vi "Update time schedule.vi"   [LabVIEW 2020]
uses:
  <vilib>/Utility/miscctls.llb/LVDateTimeRec.ctl
  Global variable.vi
types:
  T1 = typedef "LVDateTimeRec.ctl" = cluster{"fractional second":dbl, "second":i32, "minute":i32, "hour":i32, "day of month":i32, "month":i32, "year":i32, "day of week":i32, "day of year":i32, "DST":i32}
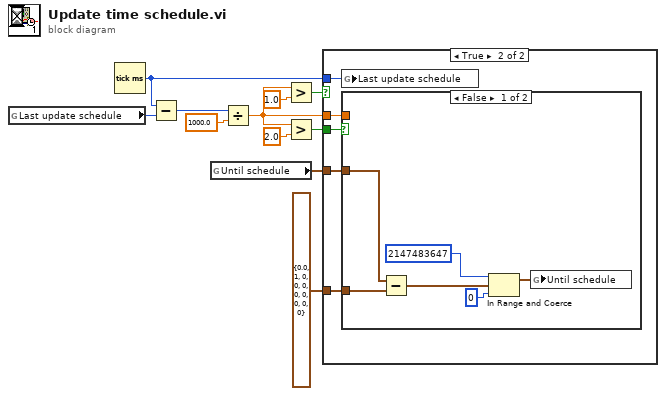
[diagram p0: block diagram]
diagram:
  n1 = global read "Global variable.vi" "Last update schedule"() -> (w11:i32)
  n2 = Tick Count (ms)() -> (millisecond timer value=w6:u32)
  n3 = Subtract(x=w6, y=w11) -> (x-y=w9:u32)
  n4 = global read "Global variable.vi" "Until schedule"() -> (w7:T1[])
  n5 = Divide(x=w9, y=1000.0) -> (x/y=w3:dbl)
  n6 = Greater?(x=w3, y=1.0) -> (0:w8:bool)
  n7 = Greater?(x=w3, y=2.0) -> (0:w4:bool)
  n8 = case shown="True" w8 {
    tunnel: w3 -> [_ w14]
    tunnel: w7 -> [_ w16]
    tunnel: w6 -> [_ w15]
    tunnel: w4 -> [_ w13]
    tunnel: T1 {"fractional second"=0.0, "second"=1, "minute"=0, "hour"=0, "day of month"=0, "month"=0, "year"=0, "day of week"=0, "day of year"=0, "DST"=0} ("t") -> [_ w12]
    frame False {
    }
    frame True {
      n9 = global write "Global variable.vi" "Last update schedule"(w15) -> ()
      n10 = case shown="False" w13 {
        tunnel: w16 -> [w19 _]
        tunnel: w14 -> [_ _]
        tunnel: w12 -> [w17 _]
        frame False {
          n11 = Subtract(x=w19, y=w17) -> (x-y=w22:T1[])
          n12 = In Range and Coerce(upper limit=2147483647, x=w22, lower limit=0) -> (coerced(x)=w18:T1[])  [unwired: 1 out]
          n13 = global write "Global variable.vi" "Until schedule"(w18) -> ()
        }
        frame True {
        }
      }
    }
  }
